vi "Process-received-message.vi"(8 "error in (no error)":errorcluster, 9 "Message":refnum<class "Message.lvclass">, 10 "Data ref. in":refnum<data-value>, 11 "UI ref. in":refnum<data-value>) -> (0 "error out":errorcluster, 2 "Data ref.":refnum<data-value>, 3 "UI ref.":refnum<data-value>)   [LabVIEW 2013, in "CameraVision.lvlib" / "CV-Main.lvclass"]
doc: "This function wraps the message checks, analysis and response action functions.\nThe validity of the message and message origin is checked, after which the appropriate module action is determined and executed.\n\nThe actions should be implemented by the module integrator."
uses:
  CV-Main.lvclass
  UI/CV-UI.lvclass
  SA-SLMAPI/Sources/Message.lvclass
  CV-Main.lvclass/CV-Main.ctl
  Read Client.vi
  Read Status.vi
  Client/Sources/CV-Client.lvclass
  SA-SLMAPI/Sources/Send-status/Send-status.lvclass
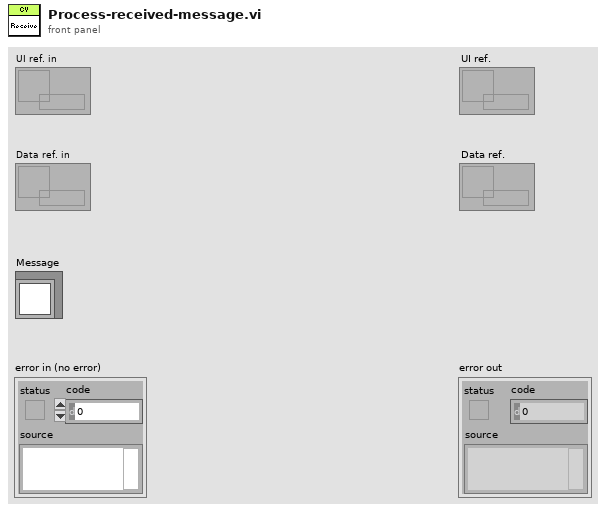
[diagram p1: front panel]
types:
  T1 = typedef "CameraVision.lvlib/CV-Client.lvclass/Supported-messages.ctl" = enum16{"Heartbeat", "Error", "Start client", "Client stopped", "Action", "Query status", "Send status", "Get clients"}
  T2 = typedef "CameraVision.lvlib/CV-Client.lvclass/Supported-modules.ctl" = enum16{"Server", "All", "SLMControl", "PowderDeposition", "StrategyParser", "CameraVision", "MaterialCharacterization", "StatusMonitor", "SLMSimulation", "LaserCharacterization"}
  T3 = typedef "CameraVision.lvlib/CV-Client.lvclass/Object-reference.ctl" = refnum<data-value>
  T4 = typedef "CameraVision.lvlib/CV-Main.lvclass/Application-states.ctl" = enum16{"Idle", "Initialized", "Configured", "Activated", "Started", "Stopped", "Reset", "Error", "Exited"}
  T5 = typedef "CameraVision.lvlib/CV-Client.lvclass/Supported-actions.ctl" = enum16{"Idle", "Initialize", "Load settings", "Load file", "Activate", "Start", "Pause", "Stop", "Repeat", "Reset", "Exit"}
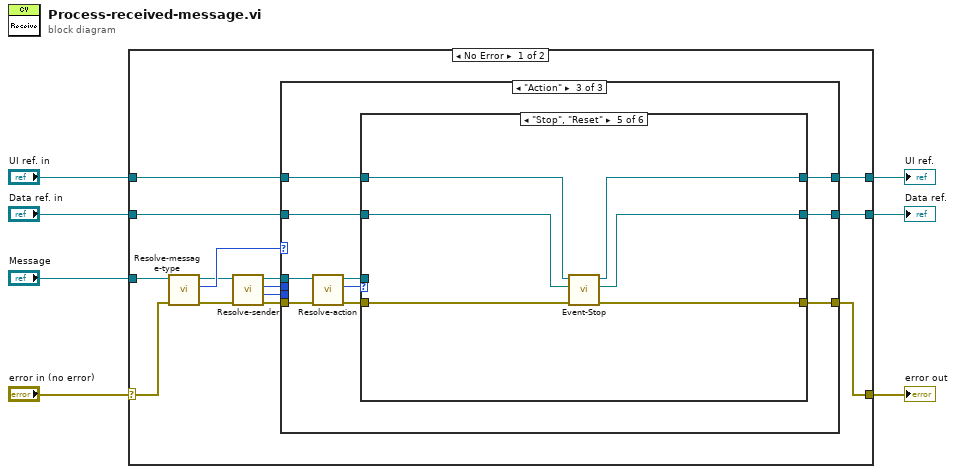
[diagram p0: block diagram]
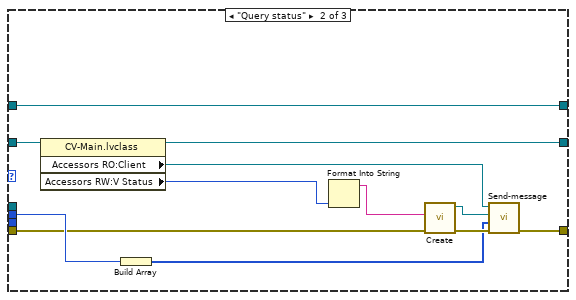
[diagram p3: hidden frame]
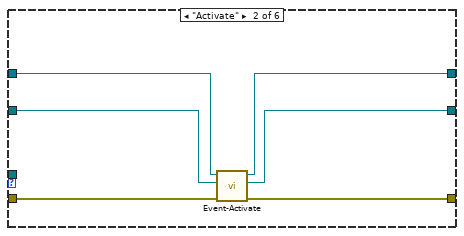
[diagram p5: hidden frame]
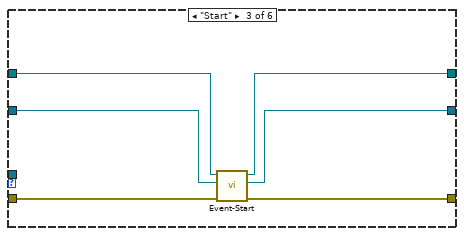
[diagram p6: hidden frame]
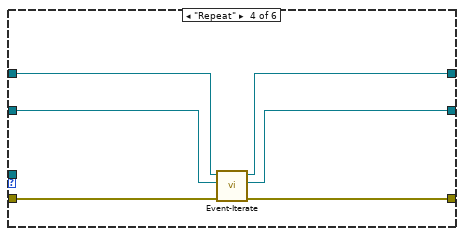
[diagram p7: hidden frame]
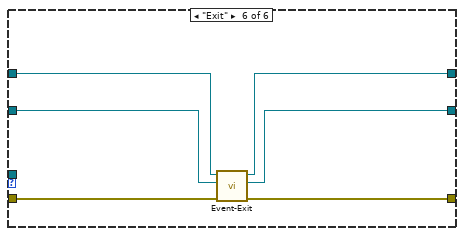
[diagram p8: hidden frame]
diagram:
  n1 = case shown="No Error" "error in (no error)" {
    selector: "error in (no error)" -> [w18 w82]
    tunnel: [w21 w82] -> w6
    tunnel: [w19 w81] -> w4
    tunnel: "UI ref. in" -> [w20 w81]
    tunnel: "Message" -> [w17 _]
    tunnel: "Data ref. in" -> [w9 w80]
    tunnel: [w8 w80] -> w1
    frame No Error {
      n2 = call "Resolve-message-type.vi"("error in (no error)"=w18, "Message"=w17) -> ("error out"=w14:errorcluster, "Message type"=w16:T1, "Message dup"=w15:refnum<class "Message.lvclass">)  [unwired: 7 in]
      n3 = call "Resolve-sender.vi"("error in (no error)"=w14, "Message"=w15) -> ("error out"=w11:errorcluster, "Sender ID"=w12:i32, "Sender type"=w13:T2, "Message dup"=w10:refnum<class "Message.lvclass">)  [unwired: 6 in]
      n4 = case shown="\"Action\"" w16 {
        tunnel: [w23 w25 w41] -> w21
        tunnel: w20 -> [w24 w36 w40]
        tunnel: [w24 w36 w38] -> w19
        tunnel: w13 -> [_ w28 _]
        tunnel: w12 -> [_ _ _]
        tunnel: w11 -> [w23 w26 w46]
        tunnel: w10 -> [_ _ w45]
        tunnel: w9 -> [w22 w35 w39]
        tunnel: [w22 w34 w37] -> w8
        frame Default {
        }
        frame "Query status" {
          n5 = property class="CV-Main.lvclass"(reference=w35) -> (reference out=w34:refnum<data-value>, "Accessors RO:Client"=w30:T3, "Accessors RW:V Status"=w31:T4)  [unwired: 1 in, 1 out]
          n6 = Build Array(w28) -> (w27:T2[])
          n7 = Format Into String(w31) -> (resulting string=w33:string)  [unwired: 3 in, 1 out]
          n8 = call "Create.vi"("error in (no error)"=w26, "Status"=w33) -> ("error out"=w29:errorcluster, "Send-status out"=w32:refnum<class "Send-status.lvclass">)  [unwired: 8 in]
          n9 = call "Send-message.vi"("error in (no error)"=w29, "Receivers"=w27, "Message"=w32, "Client in"=w30) -> ("error out"=w25:errorcluster)  [unwired: 6 in, 1 out]
        }
        frame "Action" {
          n10 = call "Resolve-action.vi"("error in (no error)"=w46, "Message"=w45) -> ("error out"=w42:errorcluster, "Action"=w43:T5, "Message dup"=w44:refnum<class "Message.lvclass">)  [unwired: 7 in]
          n11 = case shown="\"Stop\", \"Reset\"" w43 {
            tunnel: w44 -> [_ _ _ _ _ _]
            tunnel: w42 -> [w49 w51 w57 w63 w69 w75]
            tunnel: [w49 w50 w56 w62 w68 w74] -> w41
            tunnel: w40 -> [w48 w55 w61 w67 w73 w79]
            tunnel: w39 -> [w47 w52 w58 w64 w70 w76]
            tunnel: [w48 w54 w60 w66 w72 w78] -> w38
            tunnel: [w47 w53 w59 w65 w71 w77] -> w37
            frame Default {
            }
            frame "Activate" {
              n12 = call "Event-Activate.vi"("error in (no error)"=w51, "Data ref. in"=w52, "UI ref. in"=w55) -> ("error out"=w50:errorcluster, "Data ref."=w53:refnum<data-value>, "UI ref."=w54:refnum<data-value>)  [unwired: 6 in]
            }
            frame "Start" {
              n13 = call "Event-Start.vi"("error in (no error)"=w57, "Data ref. in"=w58, "UI ref. in"=w61) -> ("error out"=w56:errorcluster, "Data ref."=w59:refnum<data-value>, "UI ref."=w60:refnum<data-value>)  [unwired: 6 in]
            }
            frame "Repeat" {
              n14 = call "Event-Iterate.vi"("error in (no error)"=w63, "Data ref. in"=w64, "UI ref. in"=w67) -> ("error out"=w62:errorcluster, "Data ref."=w65:refnum<data-value>, "UI ref."=w66:refnum<data-value>)  [unwired: 6 in]
            }
            frame "Stop", "Reset" {
              n15 = call "Event-Stop.vi"("error in (no error)"=w69, "Data ref. in"=w70, "UI ref. in"=w73) -> ("error out"=w68:errorcluster, "Data ref."=w71:refnum<data-value>, "UI ref."=w72:refnum<data-value>)  [unwired: 6 in]
            }
            frame "Exit" {
              n16 = call "Event-Exit.vi"("error in (no error)"=w75, "Data ref. in"=w76, "UI ref. in"=w79) -> ("error out"=w74:errorcluster, "Data ref."=w77:refnum<data-value>, "UI ref."=w78:refnum<data-value>)  [unwired: 6 in]
            }
          }
        }
      }
    }
    frame Error {
    }
  }
  "error out" <- w6
  "UI ref." <- w4
  "Data ref." <- w1
